vi "Set 1D Array Double.vi"(5 "use temporary file? (F)":bool, 7 "column vector?":bool, 8 "error in":errorcluster, 9 "value":dbl[](array[numeric]), 10 "variable name":string, 11 "GOLPI ref. in":T1={"pipe handle"={"lv_proc.dll file path"=path "", "process instance handle"=[], "debug mode"=FALSE, "debug data"=[]}, "fast read timeout [ms]"=500, "fast read settle time [ms]"=10, "fast read to multiple [ms]"=1, "max elements per input line"=100, "slow read timeout [ms]"=5000, "stdin double format specifier"="%_16e", "max elements per stdout output column"=100, "console mode bitstream"=FALSE, "bitstream first read timeout [ms]"=1000, "bitstream read timeout [ms]"=50, "struct transfer possible"=FALSE}) -> (0 "error out":errorcluster, 3 "GOLPI ref. out":T1={"pipe handle"={"lv_proc.dll file path"=path "", "process instance handle"=[], "debug mode"=FALSE, "debug data"=[]}, "fast read timeout [ms]"=500, "fast read settle time [ms]"=10, "fast read to multiple [ms]"=1, "max elements per input line"=100, "slow read timeout [ms]"=5000, "stdin double format specifier"="%_16e", "max elements per stdout output column"=100, "console mode bitstream"=FALSE, "bitstream first read timeout [ms]"=1000, "bitstream read timeout [ms]"=50, "struct transfer possible"=FALSE})   [LabVIEW 2013, in "GOLPI library.lvlib"]
doc: "Part of polymorph Set Variable.vi"
uses:
  GOLPI library.lvlib
  Public/GOLPI reference Type Def.ctl
  LV Process source distribution/Pipe Handle.ctl
  LV Process source distribution/LV Process library.lvlib
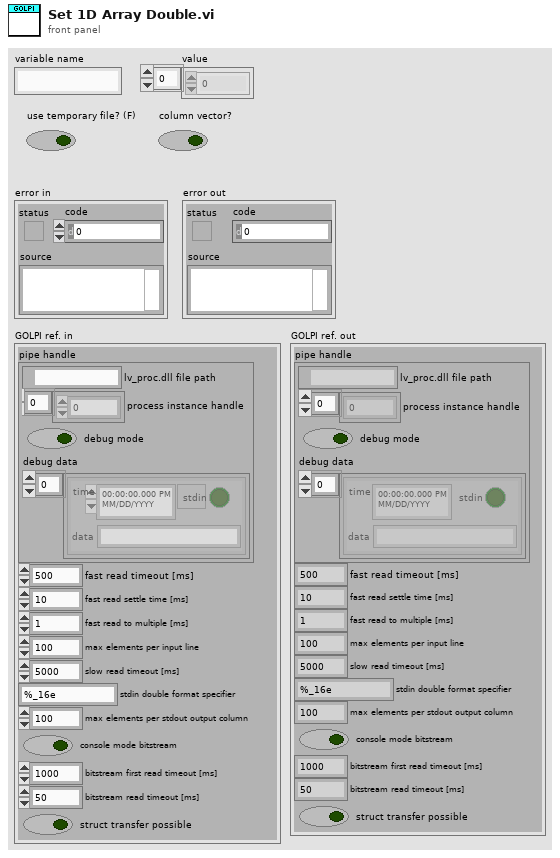
[diagram p1: front panel]
types:
  T1 = typedef "GOLPI library.lvlib/GOLPI reference Type Def.ctl" = cluster{"pipe handle":T2, "fast read timeout [ms]":u32, "fast read settle time [ms]":u32, "fast read to multiple [ms]":u32, "max elements per input line":u32, "slow read timeout [ms]":u32, "stdin double format specifier":string, "max elements per stdout output column":u32, "console mode bitstream":bool, "bitstream first read timeout [ms]":u32, "bitstream read timeout [ms]":u32, "struct transfer possible":bool}
  T2 = typedef "LV Process library.lvlib/Pipe Handle.ctl" = cluster{"lv_proc.dll file path":path, "process instance handle":u32[], "debug mode":bool, "debug data":cluster{"time":timestamp, "stdin":bool, "data":string}[]}
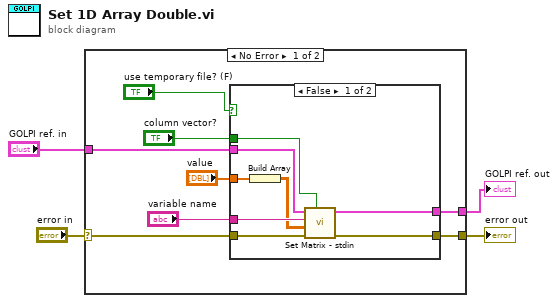
[diagram p0: block diagram]
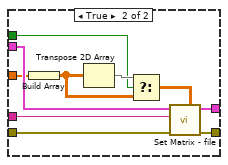
[diagram p2: hidden frame]
diagram:
  n1 = case shown="No Error" "error in" {
    selector: "error in" -> [w11 w32]
    tunnel: [w10 w32] -> w4
    tunnel: "GOLPI ref. in" -> [w9 w31]
    tunnel: [w8 w31] -> w1
    frame No Error {
      n2 = case shown="False" "use temporary file? (F)" {
        tunnel: "variable name" -> [w20 w30]
        tunnel: w11 -> [w19 w29]
        tunnel: [w18 w26] -> w10
        tunnel: w9 -> [w17 w28]
        tunnel: [w16 w27] -> w8
        tunnel: "value" -> [w15 w23]
        tunnel: "column vector?" -> [w13 w22]
        frame False {
          n3 = Build Array(w15) -> (w14:dbl[][])
          n4 = call "Set Matrix - stdin.vi"("swap dimensions? (F)"=w13, "error in"=w19, "value"=w14, "variable name"=w20, "GOLPI ref. in"=w17) -> ("error out"=w18:errorcluster, "GOLPI ref. out"=w16:T1)  [unwired: 5 in]
        }
        frame True {
          n5 = Build Array(w23) -> (w25:dbl[][])
          n6 = Transpose 2D Array(2D array=w25) -> (transposed array=w24:dbl[][])
          n7 = Select(t=w24, s=w22, f=w25) -> (s? t:f=w21:dbl[][])
          n8 = call "Set Matrix - file.vi"("double array"=w21, "error in (no error)"=w29, "variable name"=w30, "GOLPI ref. in"=w28) -> ("error out"=w26:errorcluster, "GOLPI ref. out"=w27:T1)  [unwired: 6 in]
        }
      }
    }
    frame Error {
    }
  }
  "error out" <- w4
  "GOLPI ref. out" <- w1
